vi "SingletonFGV.vi"(8 "error in (no error)":errorcluster, 11 "Destroy?":bool) -> (0 "error out":errorcluster, 3 "ServiceClientDVR":refnum<data-value>)   [LabVIEW 2019, in "MicronTemplateAPIs.lvlib" / "MicronTemplateAPIs.lvclass"]
uses:
  MicronTemplateAPIs.lvclass
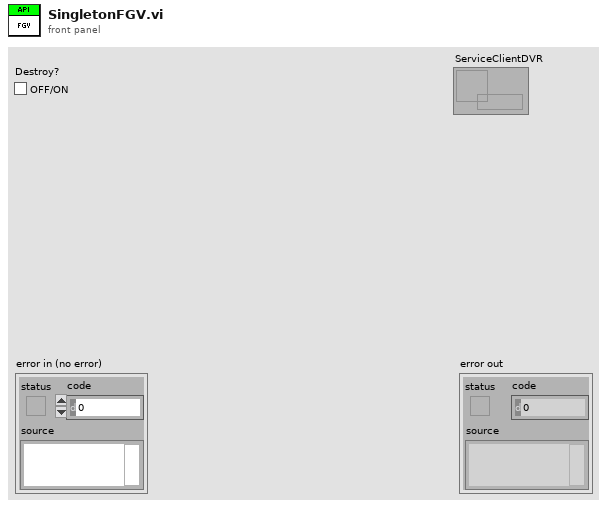
[diagram p1: front panel]
types:
  T1 = typedef "MicronClient.lvclass/ServiceDetails.ctl" = cluster{"Micron Path":path, "Network":string, "ServiceID":string, "Port":i32, "FullyQualifiedName":string, "UI":string, "Args":string, "Mode":string}
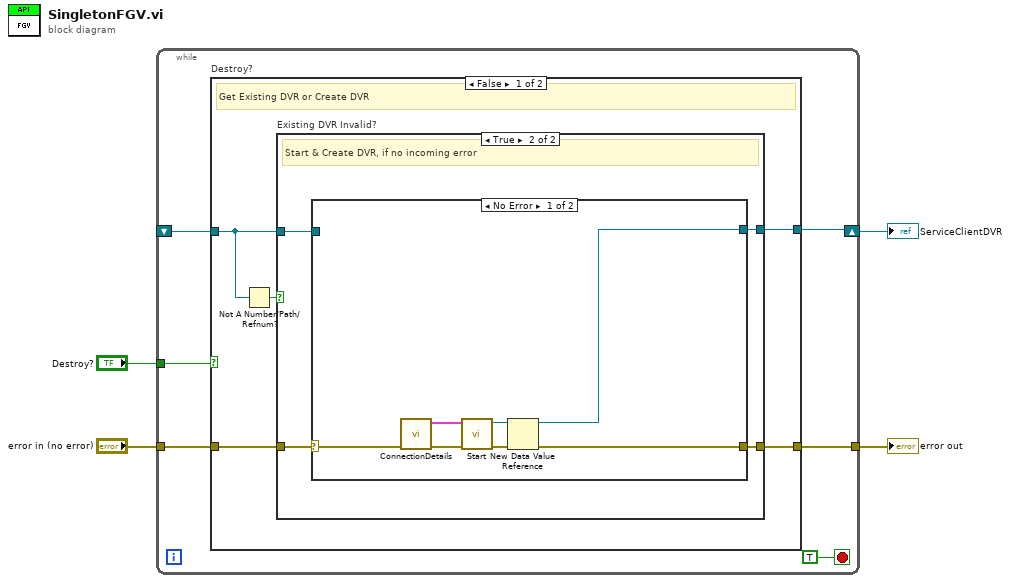
[diagram p0: block diagram]
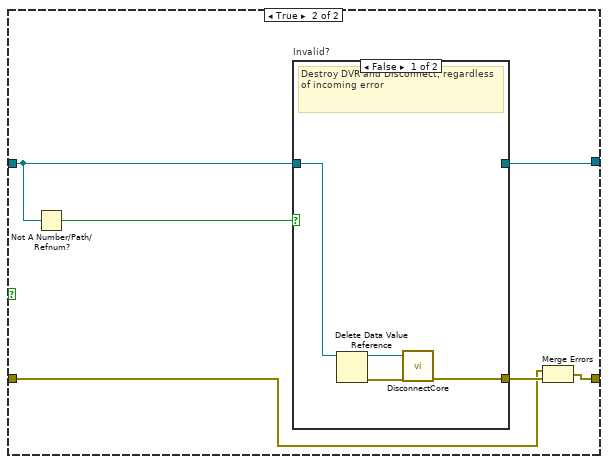
[diagram p4: hidden frame]
diagram:
  n1 = while {
    tunnel: "error in (no error)" -> [w9]
    shift-right: [w8] -> w2
    shift-left: _ -> [w7]
    tunnel: [w6] -> w3
    tunnel: "Destroy?" -> [w5]
    stop <- TRUE stop-if-true
    n2 = case "Destroy?" shown="False" w5 {
      tunnel: w9 -> [w15 w31]
      tunnel: [w14 w34] -> w8
      tunnel: w7 -> [w12 w35]
      tunnel: [w11 w32] -> w6
      frame False {
        # "Get Existing DVR or Create DVR"
        n3 = Not A Number/Path/Refnum?(number/path/refnum=w12) -> (NaN/Path/Refnum?=w13:bool)
        n4 = case "Existing DVR Invalid?" shown="True" w13 {
          tunnel: w15 -> [w16 w19]
          tunnel: [w17 w21] -> w14
          tunnel: w12 -> [w17 w18]
          tunnel: [w16 w20] -> w11
          frame False {
            # "Get Existing DVR"
          }
          frame True {
            # "Start & Create DVR, if no incoming error"
            n5 = case shown="No Error" w19 {
              selector: w19 -> [w23 w29]
              tunnel: [w26 w30] -> w21
              tunnel: [w25 w29] -> w20
              tunnel: w18 -> [_ w30]
              frame No Error {
                n6 = call "ConnectionDetails.vi"("error in (no error)"=w23) -> ("error out"=w24:errorcluster, "Connection Details"=w22:T1)  [unwired: 9 in]
                n7 = call "Start.vi"("error in (no error)"=w24, "Service Details"=w22) -> ("error out"=w28:errorcluster, "MicronTemplateAPIs out"=w27:refnum<class "MicronTemplateAPIs.lvclass">)  [unwired: 8 in]
                n8 = New Data Value Reference(data value=w27, error in=w28) -> (data value reference=w26:refnum<data-value>, error out=w25:errorcluster)
              }
              frame Error {
              }
            }
          }
        }
      }
      frame True {
        n9 = Not A Number/Path/Refnum?(number/path/refnum=w35) -> (NaN/Path/Refnum?=w36:bool)
        n10 = case "Invalid?" shown="False" w36 {
          tunnel: w35 -> [w40 w41]
          tunnel: [_ w41] -> w34
          tunnel: [w37 _] -> w33
          frame False {
            # "Destroy DVR and Disconnect, regardless of incoming error"
            n11 = Delete Data Value Reference(data value reference=w40) -> (data value=w38:refnum<class "MicronTemplateAPIs.lvclass">, error out=w39:errorcluster)  [unwired: 1 in]
            n12 = call-dynamic "DisconnectCore.vi"("error in (no error)"=w39, "GRPCClient in"=w38) -> ("error out"=w37:errorcluster)  [unwired: 8 in, 1 out]
          }
          frame True {
            # "No Action Needed"
          }
        }
        n13 = Merge Errors(w31, w33) -> (w32:errorcluster)
      }
    }
  }
  "error out" <- w3
  "ServiceClientDVR" <- w2
